vi "Actor Core.vi"(8 "error in":errorcluster, 11 "Data Viewer in":refnum<class "Accelerometer.lvclass">) -> (0 "error out":errorcluster, 3 "Actor out":refnum<class "Actor.lvclass">)   [LabVIEW 2020, in "Accelerometer.lvlib" / "Accelerometer.lvclass"]
doc: "The user interface for this panel.\n----\nCopyright: MGI 2016\nAuthor: Derek Trepanier"
uses:
  Accelerometer.lvclass
  C:/Program Files/National Instruments/LabVIEW 2020/vi.lib/MGI/Panel Manager/Panel Actor/Panel Actor/Panel Actor.lvclass
  C:/Program Files/National Instruments/LabVIEW 2020/vi.lib/ActorFramework/Actor/Actor.lvclass
  <vilib>/ActorFramework/Actor/Actor.lvclass
  Accelerometer.lvclass/Accelerometer.ctl
  <vilib>/ActorFramework/Actor/Actor.lvclass/Actor.ctl
  <vilib>/ActorFramework/Message Enqueuer/Message Enqueuer.lvclass/Message Enqueuer.ctl
  Accel task df.ctl
  <vilib>/ActorFramework/Message Enqueuer/Init from Existing Queue.vi
  <vilib>/ActorFramework/Message Enqueuer/Enqueue.vi
  <vilib>/ActorFramework/Stop Msg/Stop Msg.lvclass
  C:/Program Files/National Instruments/LabVIEW 2020/vi.lib/ActorFramework/Message/Message.lvclass
  <vilib>/ActorFramework/Message Priority Queue/Priority Enqueue.vi
  <vilib>/ActorFramework/Message Enqueuer/Message Enqueuer.lvclass
  <vilib>/MGI/Panel Manager/Panel Actor/Panel Actor/Panel Actor.lvclass
  Accelerometer Messages/Stop Trial Msg/Stop Trial Msg.lvclass
  <instrlib>/Phidgets/Phidget Accelerometer/Phidget Accelerometer.lvlib
  Accelerometer Messages/Process Live Data Q Msg/Process Live Data Q Msg.lvclass
panel:
  in  "Start Time":timestamp
  in  "Accel Task Ref":refnum<event-registration>
  in  "Accel Dev":u64[](array[numeric])
  out "Accelerometer Data":cluster{dbl, dbl, dbl, dbl}(graph)
  in  "Stop Acquire":bool
  in  "Rate Hz":u16
  in  "TDMS File Ref":refnum<k34>
  in  "Trial Num":i32
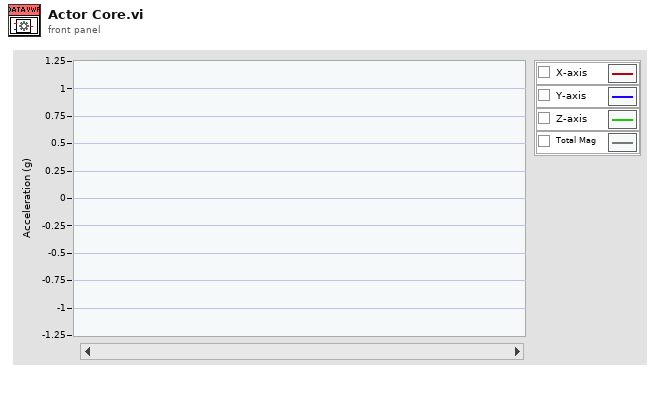
[diagram p1: front panel]
types:
  T1 = cluster{"Trial Number Update":refnum<user-event>, "Stop Acquire":refnum<user-event>, "Shut Down":refnum<user-event>, "Update Plot":refnum<user-event>}
  T2 = typedef "Accel task df.ctl" = enum16{"Idle", "Acquire", "Stop Helper Loop", "Countdown"}
  T3 = cluster{"Event Registration Refnum":refnum<event-registration>, "Pnl Actor":refnum<event-registration>}
  T4 = cluster{"X axis":dbl, "Y axis":dbl, "Z axis":dbl, "Total Mag":dbl}
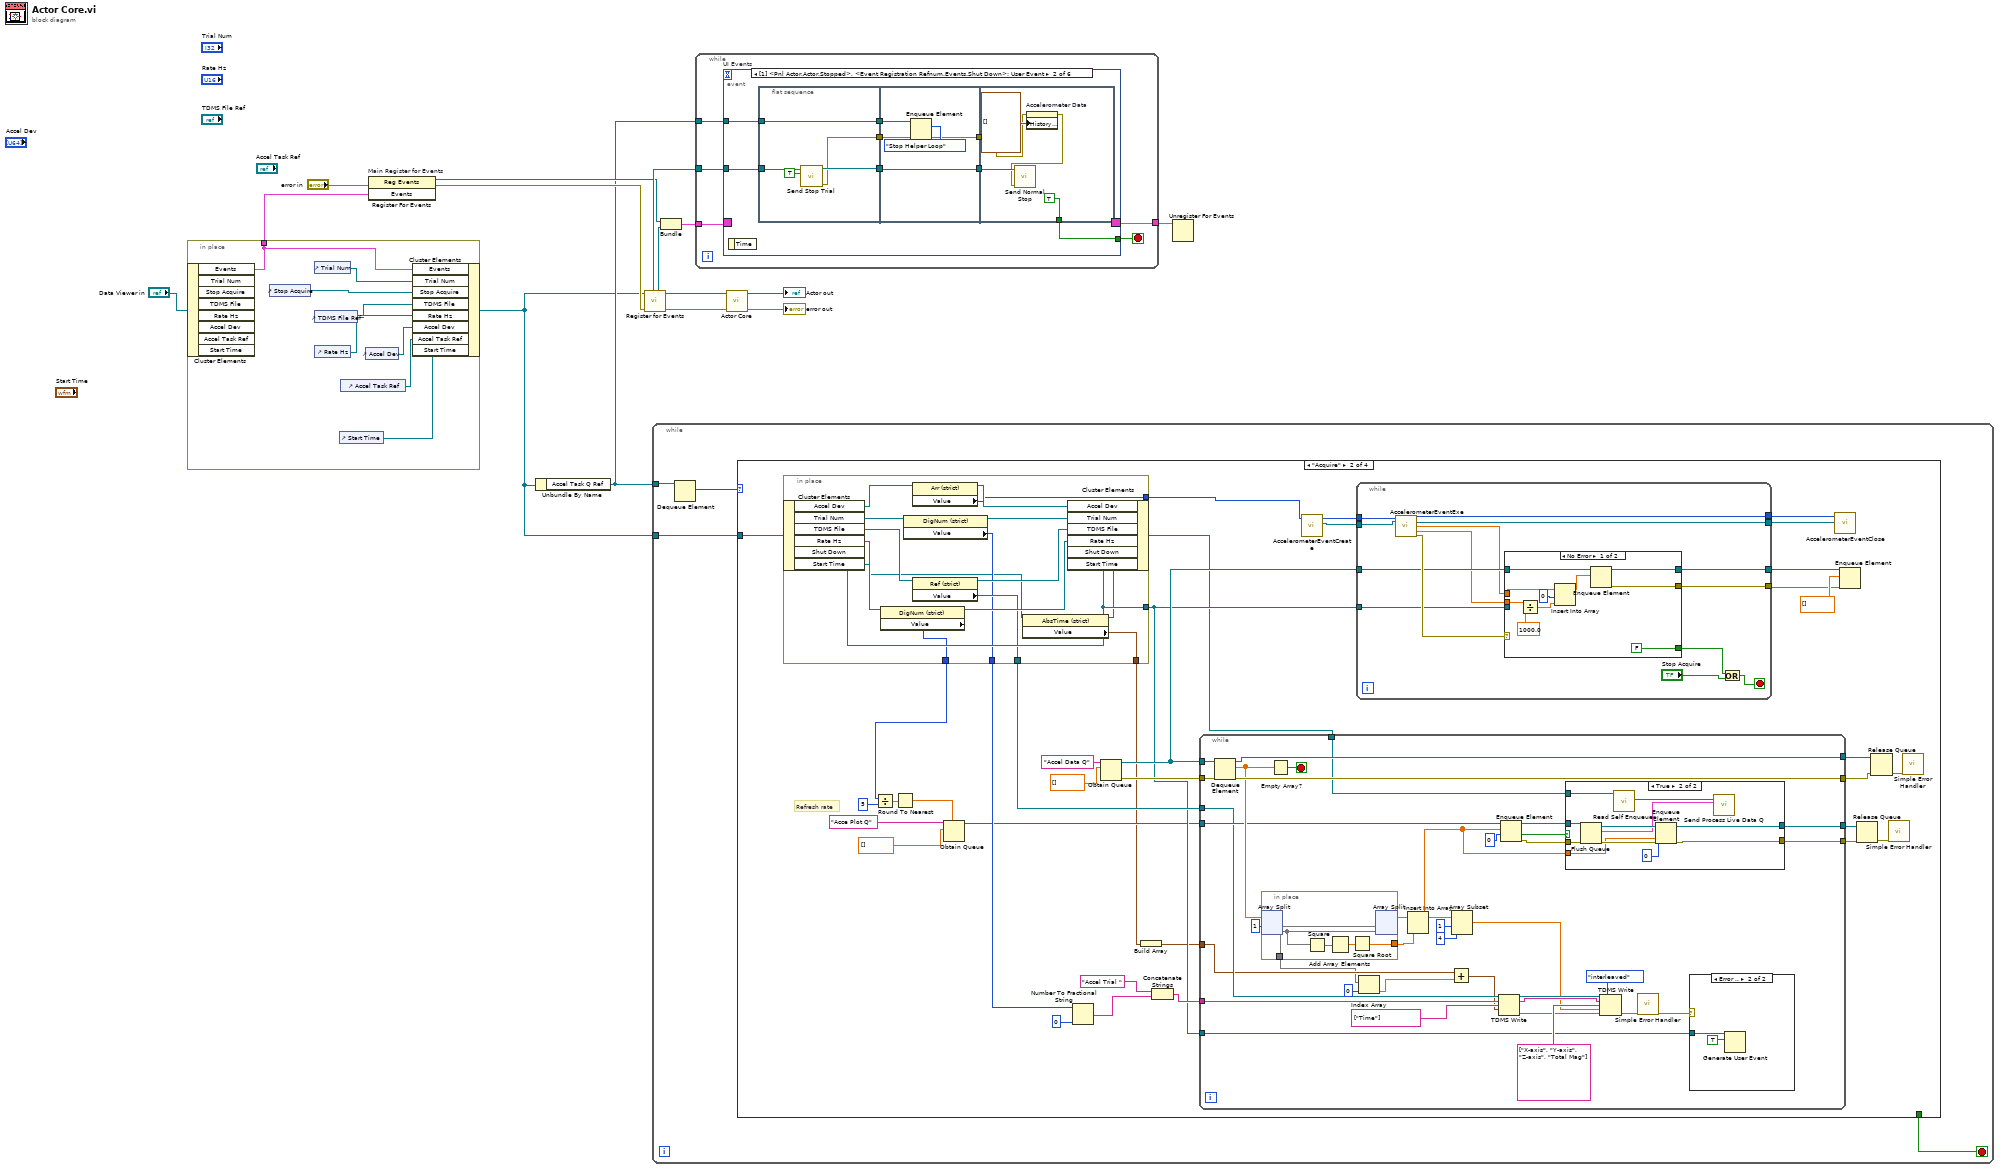
[diagram p0: block diagram]
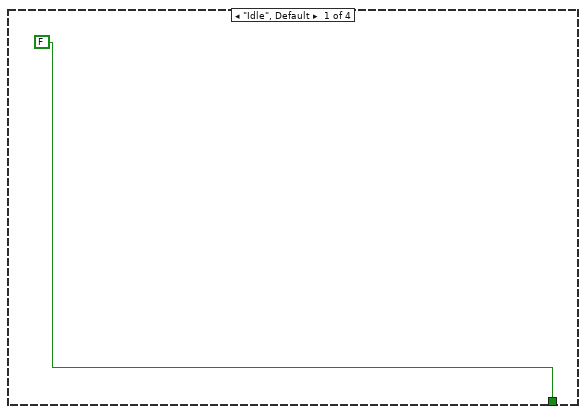
[diagram p2: hidden frame]
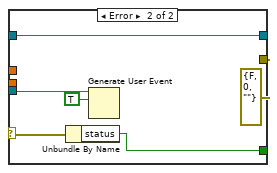
[diagram p5: hidden frame]
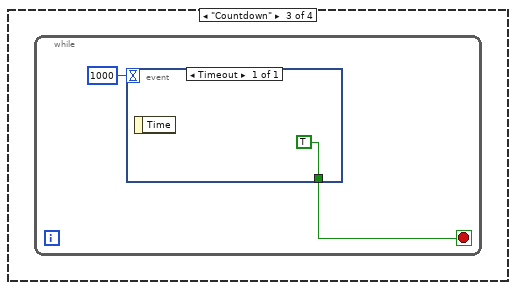
[diagram p6: hidden frame]
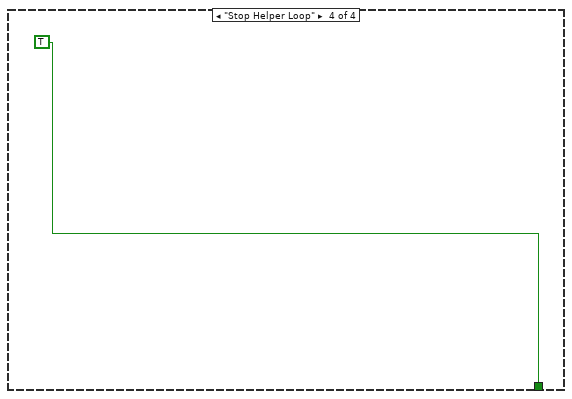
[diagram p7: hidden frame]
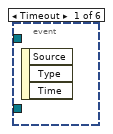
[diagram p8: hidden frame]
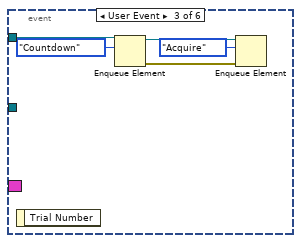
[diagram p9: hidden frame]
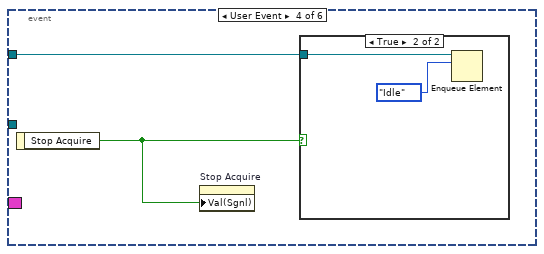
[diagram p10: hidden frame]
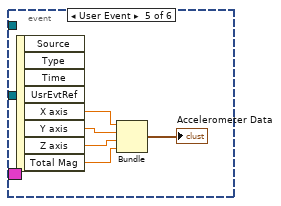
[diagram p12: hidden frame]
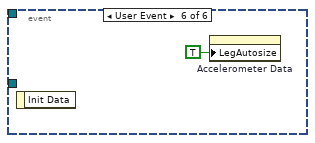
[diagram p13: hidden frame]
diagram:
  n1 = in-place {
    in-place-border: [w19] -> w9
    n2 = in-place-cluster #1("Data Viewer in") -> ("Events"=w19:T1)  [unwired: 7 out]
    n3 = control-ref of="Stop Acquire"() -> (w20:refnum<vi>)
    n4 = control-ref of="Trial Num"() -> (w21:refnum<vi>)
    n5 = control-ref of="TDMS File Ref"() -> (w22:refnum<vi>)
    n6 = control-ref of="Rate Hz"() -> (w23:refnum<vi>)
    n7 = control-ref of="Start Time"() -> (w16:refnum<vi>)
    n8 = control-ref of="Accel Task Ref"() -> (w17:refnum<vi>)
    n9 = control-ref of="Accel Dev"() -> (w18:refnum<vi>)
    n10 = in-place-cluster #1("Events"=w19, "Trial Num"=w21, "Stop Acquire"=w20, "TDMS File"=w22, "Rate Hz"=w23, "Accel Dev"=w18, "Accel Task Ref"=w17, "Start Time"=w16) -> (w1:refnum<class "Accelerometer.lvclass">)
  }
  n11 = register-events "Main Register for Events"(error in="error in", w9) -> (reference out=w6:refnum<event-registration>, error out=w5:errorcluster)  [unwired: 1 in]
  n12 = Unbundle By Name(w1) -> ("Accel Task Q Ref"=w2:refnum<queue>)
  n13 = call <vilib>:"Register for Events.vi"("Error In"=w5, "Panel Actor in"=w1) -> ("Error Out"=w13:errorcluster, "Panel Actor out"=w12:refnum<class "Accelerometer.lvclass">, "Pnl Actor"=w7:refnum<event-registration>, "Self Enqueuer"=w11:refnum<class "Message Enqueuer.lvclass">)  [unwired: 6 in]
  n14 = while {
    tunnel: w2 -> [w27]
    tunnel: w1 -> [w25]
    stop <- w24 stop-if-true
    n15 = Dequeue Element(queue=w27) -> (element=w26:T2)  [unwired: 2 in, 3 out]
    n16 = case shown="\"Acquire\"" w26 {
      tunnel: w25 -> [_ w64 _ _]
      tunnel: [FALSE _ _ TRUE] -> w24
      frame "Idle", Default {
      }
      frame "Acquire" {
        # "Refresh rate"
        n17 = in-place {
          in-place-border: [w159] -> w31
          in-place-border: [w158] -> w47
          in-place-border: [w157] -> w49
          in-place-border: [w156] -> w48
          in-place-border: [w155] -> w39
          in-place-border: [w152] -> w30
          n18 = in-place-cluster #2(w64) -> ("Accel Dev"=w161:refnum<vi>, "Trial Num"=w167:refnum<vi>, "TDMS File"=w165:refnum<vi>, "Rate Hz"=w163:refnum<vi>, "Shut Down"=w158:refnum<user-event>, "Start Time"=w154:refnum<vi>)
          n19 = property class="DigNum (strict)"(reference=w163) -> (reference out=w162:refnum<vi>, "Value"=w155:u16)  [unwired: 1 in, 1 out]
          n20 = property class="DigNum (strict)"(reference=w167) -> (reference out=w166:refnum<vi>, "Value"=w156:i32)  [unwired: 1 in, 1 out]
          n21 = property class="Arr (strict)"(reference=w161) -> (reference out=w160:refnum<vi>, "Value"=w159:u64[])  [unwired: 1 in, 1 out]
          n22 = property class="Ref (strict)"(reference=w165) -> (reference out=w164:refnum<vi>, "Value"=w157:refnum<k34>)  [unwired: 1 in, 1 out]
          n23 = property class="AbsTime (strict)"(reference=w154) -> (reference out=w153:refnum<vi>, "Value"=w152:timestamp)  [unwired: 1 in, 1 out]
          n24 = in-place-cluster #2("Accel Dev"=w160, "Trial Num"=w166, "TDMS File"=w164, "Rate Hz"=w162, "Shut Down"=w158, "Start Time"=w153) -> (w40:refnum<class "Accelerometer.lvclass">)
        }
        n25 = Divide(x=w39, y=u16 5) -> (x/y=w46:dbl)
        n26 = Round To Nearest(number=w46) -> (nearest integer value=w43:dbl)
        n27 = Obtain Queue(max queue size (-1, unlimited)=w43, name (unnamed)="Acce Plot Q", element data type=dbl[] [] ("output array")) -> (queue out=w42:refnum<queue>)  [unwired: 2 in, 2 out]
        n28 = Number To Fractional String(number=w48, precision (6)=i16 0) -> (F-format string=w53:string)  [unwired: 2 in]
        n29 = Obtain Queue(name (unnamed)="Accel Data Q", element data type=dbl[] [] ("output array")) -> (queue out=w62:refnum<queue>, error out=w56:errorcluster)  [unwired: 3 in, 1 out]
        n30 = Build Array(w30) -> (w29:timestamp[])
        n31 = Concatenate Strings("Accel Trial " ("string"), w53) -> (w50:string)
        n32 = while {
          tunnel: w62 -> [w101]
          tunnel: [w99] -> w57
          tunnel: w56 -> [w98]
          tunnel: [w97] -> w55
          tunnel: w50 -> [w77]
          tunnel: w49 -> [w76]
          tunnel: w47 -> [w90]
          tunnel: w42 -> [w87]
          tunnel: w40 -> [w86]
          tunnel: [w83] -> w38
          tunnel: [w82] -> w37
          tunnel: w29 -> [w69]
          stop <- w100 stop-if-true
          n33 = Dequeue Element(queue=w101, error in (no error)=w98) -> (queue out=w99:refnum<queue>, element=w93:dbl[], error out=w97:errorcluster)  [unwired: 1 in, 1 out]
          n34 = in-place {
            in-place-border: [w118] -> w81
            in-place-border: [w117] -> w67
            n35 = in-place-split #3(w93, 1) -> (w117:dbl[], w119:dbl[])
            n36 = Square(x=w119) -> (x^2=w121:dbl[])
            n37 = Add Array Elements(numeric array=w121) -> (sum=w120:dbl)
            n38 = Square Root(x=w120) -> (sqrt(x)=w118:dbl)
            n39 = in-place-split #3(w117, w119) -> (w80:dbl[])  [unwired: 1 out]
          }
          n40 = Empty Array?(array=w93) -> (empty?=w100:bool)
          n41 = Index Array(array=w67, index=0) -> (element=w65:dbl)
          n42 = Insert Into Array(array=w80, new element=w81) -> (w70:dbl[])  [unwired: 1 in]
          n43 = Add(x=w69, y=w65) -> (x+y=w68:timestamp[])
          n44 = Array Subset(array=w70, index=1, length=4) -> (w71:dbl[])
          n45 = TDMS Write(0:w76, 5:w77, 7:string[] ["Time"] ("channel name(s) in (Untitled)"), 9:w68) -> (4:w79:refnum<k34>, 6:w78:string, 15:w74:errorcluster)  [unwired: 2 in, 1 out]
          n46 = Enqueue Element(queue=w87, element=w70, timeout in ms (-1)=0) -> (queue out=w88:refnum<queue>, timed out?=w84:bool, error out=w85:errorcluster)  [unwired: 1 in]
          n47 = case shown="True" w84 {
            tunnel: w86 -> [_ w112]
            tunnel: [w103 w111] -> w82
            tunnel: w88 -> [w102 w109]
            tunnel: [w102 w108] -> w83
            tunnel: w85 -> [w103 w107]
            tunnel: w70 -> [_ w104]
            frame False {
            }
            frame True {
              n48 = Flush Queue(queue=w109, error in (no error)=w107) -> (queue out=w114:refnum<queue>, remaining elements=w105:cluster{"output array":dbl[]}[], error out=w113:errorcluster)
              n49 = call <vilib>:"Read Self Enqueuer.vi"("Actor"=w112) -> ("Self Enqueuer"=w106:refnum<class "Message Enqueuer.lvclass">)  [unwired: 10 in]
              n50 = Enqueue Element(queue=w114, element=w104, timeout in ms (-1)=0, error in (no error)=w113) -> (queue out=w108:refnum<queue>, error out=w111:errorcluster)  [unwired: 1 out]
              n51 = call "Send Process Live Data Q.vi"("Accel Q Elems"=w105, "Message Enqueuer in"=w106) -> ()  [unwired: 8 in, 2 out]
            }
          }
          n52 = TDMS Write(0:w79, 1:enum16{"decimated", "interleaved"}."interleaved" ("data layout (0:decimated)"), 5:w78, 7:string[] ["X-axis", "Y-axis", "Z-axis", "Total Mag"] ("channel name(s) in (Untitled)"), 9:w71, 11:w74) -> (15:w95:errorcluster)  [unwired: 3 out]
          n53 = call <vilib>:"Simple Error Handler.vi"("error in (no error)"=w95) -> ("error out"=w91:errorcluster)  [unwired: 4 in, 4 out]
          n54 = case shown="Error .." w91 {
            tunnel: w90 -> [_ w116]
            frame No Error {
            }
            frame Error {
              n55 = Generate User Event(user event=w116, event data cluster=TRUE ("event data")) -> ()  [unwired: 2 in, 2 out]
            }
          }
        }
        n56 = call <instrlib>:"AccelerometerEventCreate.vi"("Devices In"=w31) -> ("Event Registration Refnum"=w32:refnum<event-registration>, "Devices Out"=w33:u64[])  [unwired: 8 in, 1 out]
        n57 = while {
          tunnel: w33 -> [w135]
          tunnel: w62 -> [w133]
          tunnel: [w130] -> w58
          tunnel: [w129] -> w60
          tunnel: w47 -> [w126]
          tunnel: [w125] -> w35
          tunnel: [w124] -> w34
          tunnel: w32 -> [w122]
          stop <- w128 stop-if-true
          n58 = call <instrlib>:"AccelerometerEventExe.vi"("Devices In"=w135, "Event Registration Refnum In"=w122) -> ("Devices Out"=w124:u64[], "Event Registration Refnum Out"=w125:refnum<event-registration>, "Accel Data"=w131:dbl[], "Timestamp"=w132:dbl, "error out"=w134:errorcluster)  [unwired: 6 in, 3 out]
          n59 = case shown="No Error" w134 {
            selector: w134 -> [_ w147]
            tunnel: w133 -> [w145 w150]
            tunnel: w132 -> [w138 _]
            tunnel: w131 -> [w144 _]
            tunnel: [w141 errorcluster {"status"=FALSE, "code"=0, "source"=""} ("error out")] -> w130
            tunnel: [w140 w150] -> w129
            tunnel: [FALSE w146] -> w127
            tunnel: w126 -> [_ w149]
            frame No Error {
              n60 = Divide(x=w138, y=1000.0) -> (x/y=w137:dbl)
              n61 = Insert Into Array(array=w144, index=0, new element=w137) -> (w142:dbl[])
              n62 = Enqueue Element(queue=w145, element=w142) -> (queue out=w140:refnum<queue>, error out=w141:errorcluster)  [unwired: 2 in, 1 out]
            }
            frame Error {
              n63 = Unbundle By Name(w147) -> ("status"=w146:bool)
              n64 = Generate User Event(user event=w149, event data cluster=TRUE ("event data")) -> ()  [unwired: 2 in, 2 out]
            }
          }
          n65 = Or(x=w127, y="Stop Acquire") -> (x .or. y?=w128:bool)
        }
        n66 = call <instrlib>:"AccelerometerEventClose.vi"("Event Registration Refnum In"=w35, "Devices In"=w34) -> ()  [unwired: 8 in, 2 out]
        n67 = Enqueue Element(queue=w60, element=dbl[] [] ("output array"), error in (no error)=w58) -> ()  [unwired: 1 in, 3 out]
        n68 = Release Queue(queue=w38, error in (no error)=w37) -> (error out=w36:errorcluster)  [unwired: 1 in, 2 out]
        n69 = Release Queue(queue=w57, error in (no error)=w55) -> (error out=w54:errorcluster)  [unwired: 1 in, 2 out]
        n70 = call <vilib>:"Simple Error Handler.vi"("error in (no error)"=w36) -> ()  [unwired: 4 in, 5 out]
        n71 = call <vilib>:"Simple Error Handler.vi"("error in (no error)"=w54) -> ()  [unwired: 4 in, 5 out]
      }
      frame "Countdown" {
        n72 = while {
          stop <- w168 stop-if-true
          n73 = event shown="[0] Timeout" {
            selector: _ -> [_]
            dyn-events: _ -> [_]
            timeout: 1000 -> [_]
            tunnel: [TRUE] -> w168
            event Timeout {
              n74 = event-data() -> ()  [unwired: 1 in, 1 out]
            }
          }
        }
      }
      frame "Stop Helper Loop" {
      }
    }
  }
  n75 = Bundle("Event Registration Refnum"=w6, "Pnl Actor"=w7) -> (w4:T3)  [unwired: 1 in]
  n76 = while {
    tunnel: w11 -> [w175]
    tunnel: w4 -> [w174]
    tunnel: [w173] -> w3
    tunnel: w2 -> [w172]
    stop <- w176 stop-if-true
    n77 = event "UI Events" shown="[1] <Pnl Actor.Actor.Stopped>, <Event Registration Refnum.Events.Shut Down>: User Event" {
      selector: w174 -> [_ _ _ _ _ _]
      dyn-events: [_ _ _ _ _ _] -> w173
      timeout: _ -> [_ _ _ _ _ _]
      tunnel: [_ w179 _ _ _ _] -> w176
      tunnel: w175 -> [_ w182 _ _ _ _]
      tunnel: w172 -> [_ w183 w204 w205 _ _]
      event Timeout {
        n78 = event-data() -> ()  [unwired: 1 in, 3 out]
      }
      event User Event {
        n79 = event-data() -> ()  [unwired: 1 in, 1 out]
        n80 = flat-sequence {
          tunnel: [w189] -> w184
          tunnel: w183 -> [w189]
          tunnel: w182 -> [w188]
          tunnel: [w187] -> w180
          tunnel: [w185] -> w178
          tunnel: w184 -> [w194]
          tunnel: [w192] -> w181
          tunnel: w180 -> [w192]
          tunnel: w178 -> [w191]
          tunnel: [w190] -> w177
          tunnel: w181 -> [w199]
          tunnel: [TRUE] -> w179
          tunnel: w177 -> [w196]
          frame #0 {
            n81 = call "Send Stop Trial.vi"("Stop Acquiring"=TRUE, "Message Enqueuer in"=w188) -> ("error out"=w185:errorcluster, "Message Enqueuer out"=w187:refnum<class "Message Enqueuer.lvclass">)  [unwired: 8 in]
          }
          frame #1 {
            n82 = Enqueue Element(queue=w194, element=Accel_task_df."Stop Helper Loop", error in (no error)=w191) -> (error out=w190:errorcluster)  [unwired: 1 in, 2 out]
          }
          frame #2 {
            n83 = property on="Accelerometer Data" class="WFChart (strict)"(error in=w196, "History Data"=cluster{dbl, dbl, dbl, dbl}[] []) -> (error out=w195:errorcluster)  [unwired: 1 in, 1 out]
            n84 = call <vilib>:"Send Normal Stop.vi"("error in (no error)"=w195, "Message Enqueuer"=w199) -> ()  [unwired: 9 in, 1 out]
          }
        }
      }
      event User Event {
        n85 = event-data() -> ()  [unwired: 1 in, 1 out]
        n86 = Enqueue Element(queue=w204, element=Accel_task_df."Countdown") -> (queue out=w202:refnum<queue>, error out=w201:errorcluster)  [unwired: 2 in, 1 out]
        n87 = Enqueue Element(queue=w202, element=Accel_task_df."Acquire", error in (no error)=w201) -> ()  [unwired: 1 in, 3 out]
      }
      event User Event {
        n88 = event-data() -> ("Stop Acquire"=w206:bool)  [unwired: 1 in]
        n89 = property on="Stop Acquire" class="Bool (strict)"("Val(Sgnl)"=w206) -> ()  [unwired: 2 in, 2 out]
        n90 = case shown="True" w206 {
          tunnel: w205 -> [_ w208]
          frame False {
          }
          frame True {
            n91 = Enqueue Element(queue=w208, element=Accel_task_df."Idle") -> ()  [unwired: 2 in, 3 out]
          }
        }
      }
      event User Event {
        n92 = event-data() -> ("X axis"=w213:dbl, "Y axis"=w212:dbl, "Z axis"=w210:dbl, "Total Mag"=w211:dbl)  [unwired: 1 in, 4 out]
        n93 = Bundle("X axis"=w213, "Y axis"=w212, "Z axis"=w210, "Total Mag"=w211) -> (→"Accelerometer Data":T4)  [unwired: 1 in]
      }
      event User Event {
        n94 = event-data() -> ()  [unwired: 1 in, 1 out]
        n95 = property on="Accelerometer Data" class="WFChart (strict)"("LegAutosize"=TRUE ("Legend:Autosize")) -> ()  [unwired: 2 in, 2 out]
      }
    }
  }
  n96 = call-parent "Actor Core.vi"("error in"=w13, "Panel Actor in"=w12) -> ("error out"=→"error out":errorcluster, "Actor out"=→"Actor out":refnum<class "Actor.lvclass">)  [unwired: 8 in]
  n97 = Unregister For Events(event registration refnum=w3) -> ()  [unwired: 1 in, 1 out]
